vi "DSF.Engine.Framework.Shutdown.vi"(8 "error in (no error)":errorcluster, 11 "Framework in":refnum<class "DSF.Engine.Framework.lvclass">) -> (0 "error out":errorcluster, 3 "Framework out":refnum<class "DSF.Engine.Framework.lvclass">)   [LabVIEW 2017, in "Data Sharing Framework Engine.lvlib" / "DSF.Engine.Framework.lvclass"]
uses:
  DSF.Engine.Framework.lvclass
  DSF.Engine.Framework.lvclass/DSF.Engine.Framework.ctl
  Transceiver/DSF.Engine.Transceiver.lvclass
  Plugin/DSF.Engine.Plugin.lvclass
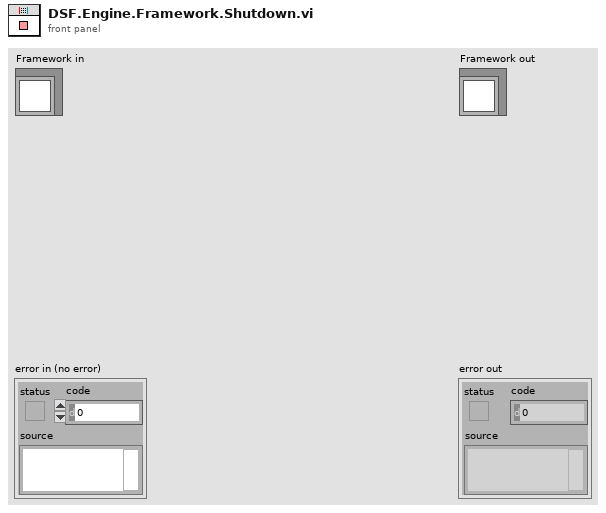
[diagram p1: front panel]
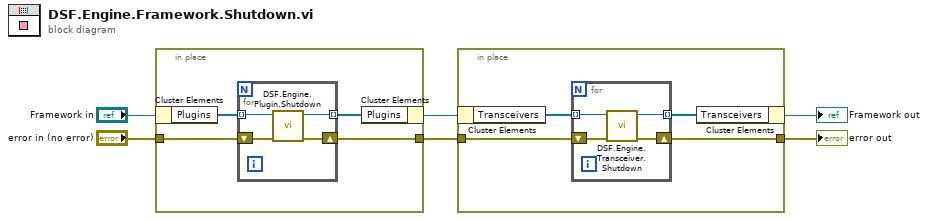
[diagram p0: block diagram]
diagram:
  n1 = in-place {
    in-place-border: "error in (no error)" -> [w10]
    in-place-border: [w9] -> w4
    n2 = in-place-cluster #1("Framework in") -> ("Plugins"=w8:refnum<class "DSF.Engine.Plugin.lvclass">[])
    n3 = for {
      tunnel: w8 -> [w11] mode=indexing
      tunnel: [w12] -> w7 mode=indexing
      shift-right: [w13] -> w9
      shift-left: w10 -> [w14]
      n4 = call "DSF.Engine.Plugin.Shutdown.vi"("error in (no error)"=w14, "Plugin in"=w11) -> ("error out"=w13:errorcluster, "Plugin out"=w12:refnum<class "DSF.Engine.Plugin.lvclass">)  [unwired: 8 in]
    }
    n5 = in-place-cluster #1("Plugins"=w7) -> (w3:refnum<class "DSF.Engine.Framework.lvclass">)
  }
  n6 = in-place {
    in-place-border: w4 -> [w18]
    in-place-border: [w17] -> w2
    n7 = in-place-cluster #2(w3) -> ("Transceivers"=w16:refnum<class "DSF.Engine.Transceiver.lvclass">[])
    n8 = for {
      tunnel: w16 -> [w22] mode=indexing
      shift-right: [w20] -> w17
      shift-left: w18 -> [w21]
      tunnel: [w19] -> w15 mode=indexing
      n9 = call-dynamic "DSF.Engine.Transceiver.Shutdown.vi"("error in (no error)"=w21, "Transceiver in"=w22) -> ("error out"=w20:errorcluster, "Transceiver out"=w19:refnum<class "DSF.Engine.Transceiver.lvclass">)  [unwired: 8 in]
    }
    n10 = in-place-cluster #2("Transceivers"=w15) -> (→"Framework out":refnum<class "DSF.Engine.Framework.lvclass">)
  }
  "error out" <- w2
